vi "Current Sensor Driver.vi"(8 "VSupply":fxp<+/-,24,5>, 9 "IRange":fxp<+,27,10>, 11 "VInput":fxp<+/-,26,5>) -> (2 "ISensor":fxp<+/-,19,15>, 3 "bSensorOK":bool)   [LabVIEW 2015]
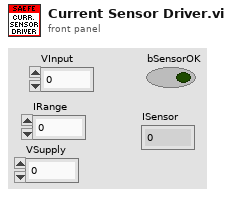
[diagram p1: front panel]
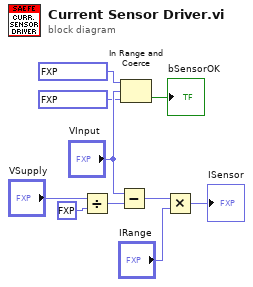
[diagram p0: block diagram]
diagram:
  n1 = Divide(x="VSupply", y=fxp<+/-,26,5> 2.0) -> (x/y=w1:fxp<+/-,24,4>)
  n2 = Subtract(x="VInput", y=w1) -> (x-y=w9:fxp<+/-,24,5>)
  n3 = In Range and Coerce(upper limit=fxp<+/-,14,5> 4.599609375, x="VInput", lower limit=fxp<+/-,14,5> 0.400390625) -> (In Range?=→"bSensorOK":bool)  [unwired: 1 out]
  n4 = Multiply(x=w9, y="IRange") -> (x*y=→"ISensor":fxp<+/-,19,15>)
